vi "Configuration Viewer.vi"() -> ()   [LabVIEW 2012]
uses:
  Configuration/_Global Configuration.vi
panel:
  out "Restore From Power Failure":bool
  out "Enable Voltage Reset":bool=TRUE
  out "Table":i32(listbox)=-1
  in  "Export Config":bool
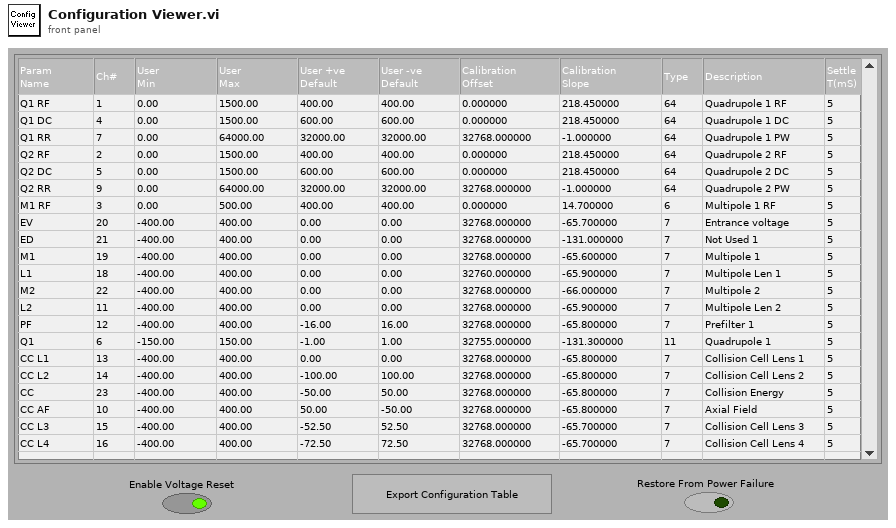
[diagram p1: front panel]
types:
  T1 = enum32{"existing file", "new file", "new or existing file", "existing dir", "new dir", "new or existing dir", "existing file (use LLBs)", "new file (use LLBs)", "new or existing file (use LLBs)", "new or existing file or directory (use LLBs)"}
  T2 = typedef "_RT Instrument 2.ctl" = cluster{"Table":T3[], "Instrument":string[]}
  T3 = typedef "_RT Configuration 2.ctl" = cluster{"Name":string, "Ch#":u8, "Min":dbl, "Max":dbl, "Def+":dbl, "Def-":dbl, "Offset":dbl, "Slope":dbl, "Type":u8, "Description":string, "SettleT":dbl}
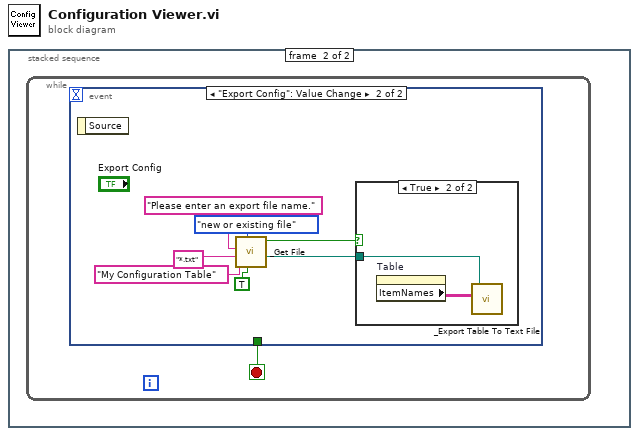
[diagram p0: block diagram]
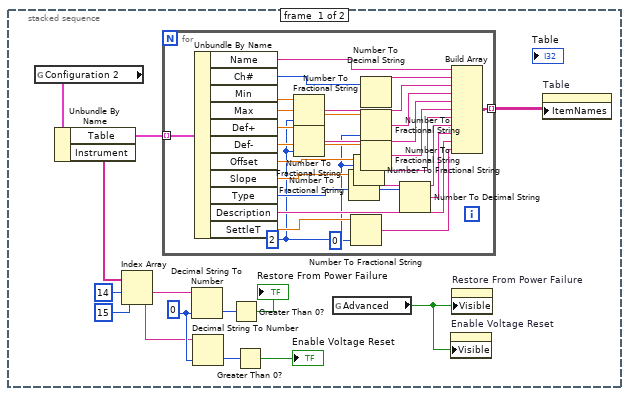
[diagram p2: hidden frame]
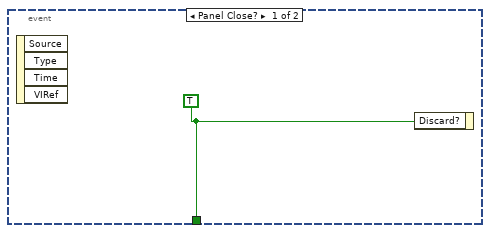
[diagram p3: hidden frame]
diagram:
  n1 = stacked-sequence {
    frame #0 {
      w3 = 0 ("default (0 I32)")
      n2 = global read "_Global Configuration.vi" "Configuration 2"() -> (w14:T2)
      n3 = Unbundle By Name(w14) -> ("Table"=w13:T3[], "Instrument"=w11:string[])
      n4 = Index Array(array=w11, index #1=14 ("index"), index #2=15 ("index")) -> (element #1=w7:string, element #2=w1:string)
      n5 = for {
        tunnel: w13 -> [w38] mode=indexing
        tunnel: [w25] -> w12 mode=indexing
        w16 = i16 2 ("precision (6)")
        n6 = Unbundle By Name(w38) -> ("Name"=w24:string, "Ch#"=w37:u8, "Min"=w35:dbl, "Max"=w34:dbl, "Def+"=w33:dbl, "Def-"=w32:dbl, "Offset"=w31:dbl, "Slope"=w23:dbl, "Type"=w21:u8, "Description"=w19:string, "SettleT"=w18:dbl)
        n7 = Number To Fractional String(number=w35, precision (6)=w16) -> (F-format string=w30:string)  [unwired: 2 out]
        n8 = Number To Fractional String(number=w33, precision (6)=w16) -> (F-format string=w28:string)  [unwired: 2 out]
        n9 = Number To Fractional String(number=w23) -> (F-format string=w22:string)  [unwired: 3 out]
        n10 = Number To Fractional String(number=w18, precision (6)=i16 0) -> (F-format string=w17:string)  [unwired: 2 out]
        n11 = Number To Fractional String(number=w31) -> (F-format string=w26:string)  [unwired: 3 out]
        n12 = Number To Decimal String(number=w37) -> (decimal integer string=w36:string)  [unwired: 1 out]
        n13 = Number To Fractional String(number=w34, precision (6)=w16) -> (F-format string=w29:string)  [unwired: 2 out]
        n14 = Number To Fractional String(number=w32, precision (6)=w16) -> (F-format string=w27:string)  [unwired: 2 out]
        n15 = Number To Decimal String(number=w21) -> (decimal integer string=w20:string)  [unwired: 1 out]
        n16 = Build Array(w24, w36, w30, w29, w28, w27, w26, w22, w20, w19, w17) -> (w25:string[])
      }
      n17 = Decimal String To Number(string=w7, default (0L)=w3) -> (number=w8:i32)  [unwired: 2 out]
      n18 = Decimal String To Number(string=w1, default (0L)=w3) -> (number=w4:i32)  [unwired: 2 out]
      n19 = Greater Than 0?(x=w8) -> (x > 0?=→"Restore From Power Failure":bool)
      n20 = Greater Than 0?(x=w4) -> (x > 0?=→"Enable Voltage Reset":bool)
      n21 = global read "_Global Configuration.vi" "Advanced"() -> (w10:bool)
      n22 = property on="Enable Voltage Reset" class="Bool (strict)"("Visible"=w10) -> ()  [unwired: 2 in, 2 out]
      n23 = property on="Restore From Power Failure" class="Bool (strict)"("Visible"=w10) -> ()  [unwired: 2 in, 2 out]
      n24 = property on="Table" class="MCListbox (strict)"("ItemNames"=w12) -> ()  [unwired: 2 in, 2 out]
    }
    frame #1 {
      n25 = while {
        stop <- w39 stop-if-true
        n26 = event shown="[1] \"Export Config\": Value Change" {
          selector: _ -> [_ _]
          dyn-events: _ -> [_ _]
          timeout: _ -> [_ _]
          tunnel: [w40 _] -> w39
          event Panel Close? {
            w40 = TRUE
            n27 = event-data() -> ()  [unwired: 5 out]
            n28 = event-data("Discard?"=w40) -> ()  [unwired: 1 in, 1 out]
          }
          event "Export Config": Value Change {
            n29 = event-data() -> ()  [unwired: 2 out]
            n30 = call "_Get File.vi"("For Write (T)"=TRUE, "select mode (new or existing)"=T1."new or existing file", "default name"="My Configuration Table", "extension (isd)"="*.txt" ("pattern (all files)"), "prompt"="Please enter an export file name.") -> ("Seleted File"=w41:path, "Succeeded"=w42:bool)  [unwired: 1 in, 2 out]
            n31 = case shown="True" w42 {
              tunnel: w41 -> [_ w48]
              frame False {
              }
              frame True {
                n32 = property on="Table" class="MCListbox (strict)"() -> ("ItemNames"=w49:string[][])  [unwired: 2 in, 2 out]
                n33 = call "_Export Table To Text File.vi"("2D data"=w49, "file path (dialog if empty)"=w48) -> ()  [unwired: 4 in, 3 out]
              }
            }
          }
        }
      }
    }
  }
